vi "SwerveKinematics.vi"(0 "Joystick X":dbl(slide) scale=-1.0..1.0, 2 "Saturation Velocity (ul)":dbl=1.0, 5 "Joystick Y":dbl(slide) scale=1.0..-1.0, 7 "Joystick Rotation":dbl(slide) scale=1.0..-1.0, 9 "Cx (in)":dbl, 11 "Cy (in)":dbl) -> (1 "Module 0 Angle (deg)":dbl(knob) scale=180.0..-180.0 scale format="%#_6f", 3 "Module 1 Angle (deg)":dbl(knob) scale=180.0..-180.0 scale format="%#_6f", 4 "Module 0 Velocity Command (ul)":dbl(slide) scale=0.0..1.0 scale format="%.2f", 6 "Module 1 Velocity Command (ul)":dbl(slide) scale=0.0..1.0 scale format="%.2f", 10 "Module 2 Velocity Command (ul)":dbl(slide) scale=0.0..1.0 scale format="%.2f", 12 "Module 3 Angle (deg)":dbl(knob) scale=180.0..-180.0 scale format="%#_6f", 14 "Module 2 Angle (deg)":dbl(knob) scale=180.0..-180.0 scale format="%#_6f", 15 "Module 3 Velocity Command (ul)":dbl(slide) scale=0.0..1.0 scale format="%.2f")   [LabVIEW 2020]
doc: "Performs the kinematics for a rectangular four wheel swerve robot with a selectable center of rotation. Swerve module #0 is located in the front right corner and the modules increment in the counter-clockwise direction. This VI also handles de-saturating the drive velocity commands."
uses:
  GlobalDrivebase.vi
panel:
  # "\"Front\" of Robot"
  # "M1"
  # "M0"
  # "Left Thumbstick"
  # "Right Thumbstick"
  # "X"
  # "Y"
  # "(0,0)"
  # "+CCW"
  # "M2"
  # "M3"
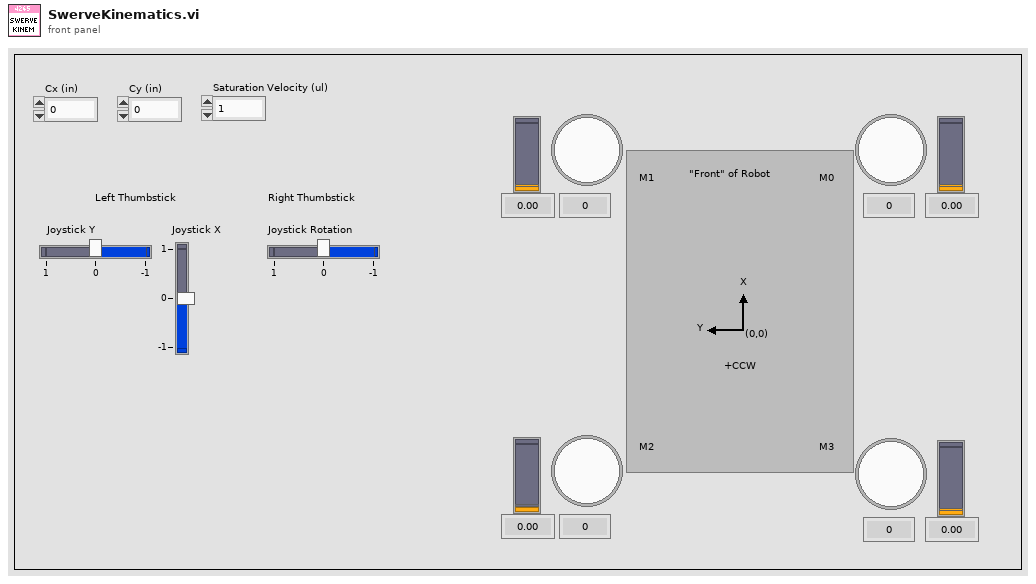
[diagram p1: front panel]
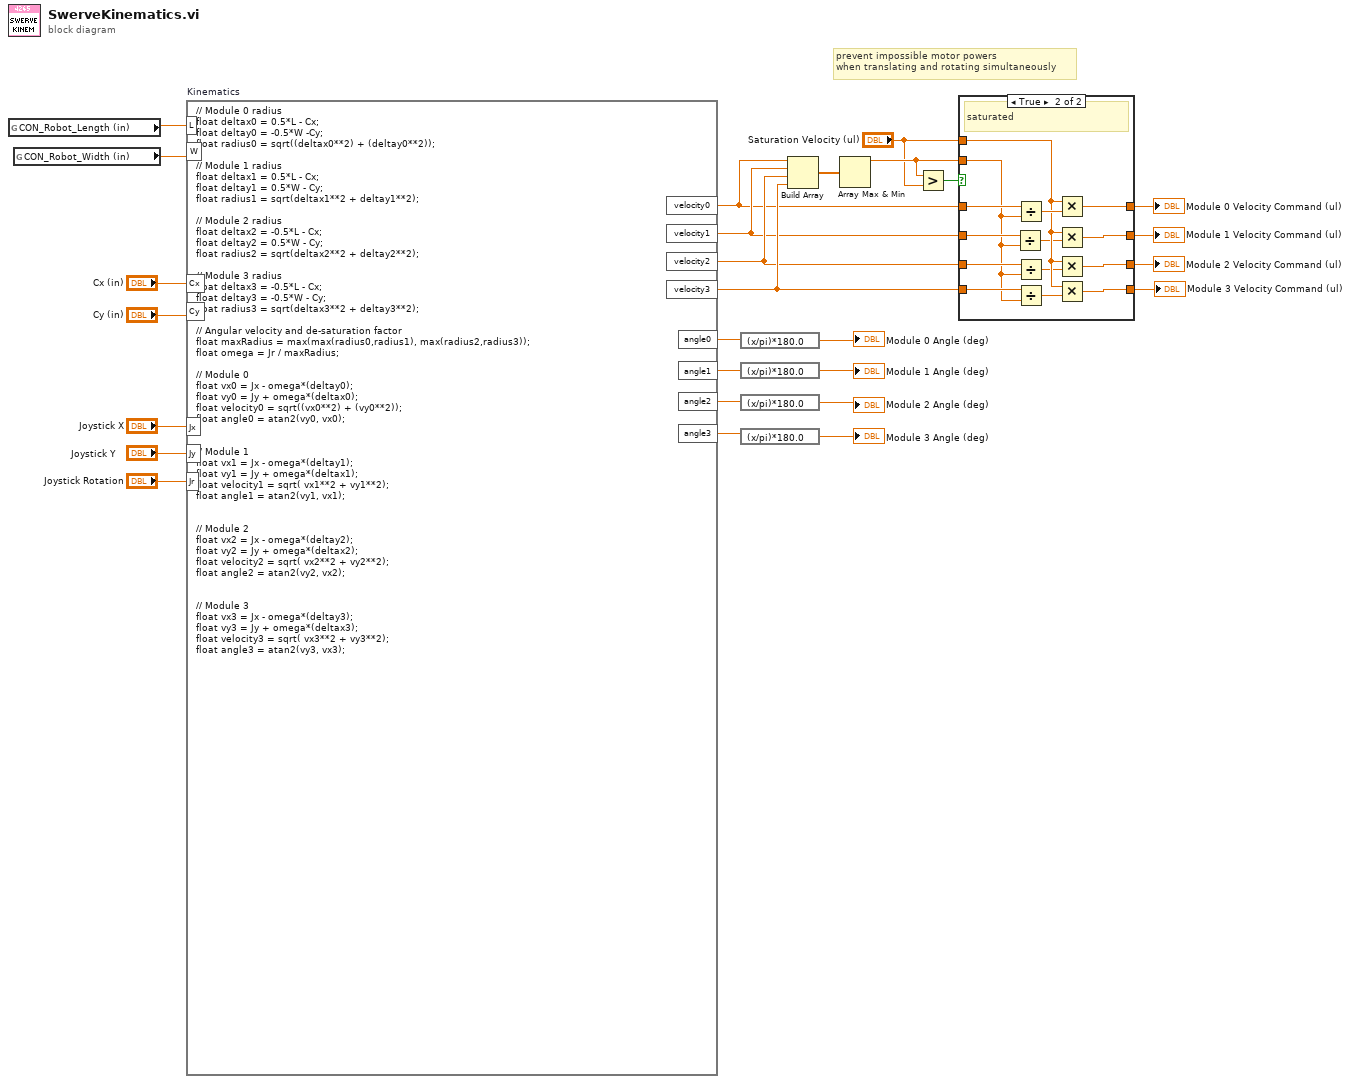
[diagram p0: block diagram]
diagram:
  # "prevent impossible motor powers\nwhen translating and rotating simultaneously"
  n1 = global read "GlobalDrivebase.vi" "CON_Robot_Length (in)"() -> (w2:dbl)
  n2 = global read "GlobalDrivebase.vi" "CON_Robot_Width (in)"() -> (w1:dbl)
  n3 = formula code="// Module 0 radius\nfloat deltax0 = 0.5*L - Cx;\nfloat deltay0 = -0.5*W -Cy; \nfloat radius0 = sqrt((deltax0**2) + (deltay0**2));\n\n// Module 1 radius\nfloat deltax1 = 0.5*L - Cx;\nfloat deltay1 = 0.5*W - Cy;\nfloat radius1 = sqrt(deltax1**2 + deltay1**2);\n\n// Module 2 radius\nfloat deltax2 = -0.5*L - Cx;\nfloat deltay2 = 0.5*W - Cy;\nfloat radius2 = sqrt(deltax2**2 + deltay2**2);\n\n// Module 3 radius\nfloat deltax3 = -0.5*L - Cx;\nfloat deltay3 = -0.5*W - Cy;\nfloat radius3 = sqrt(deltax3**2 + deltay3**2);\n\n// Angular velocity and de-saturation factor\nfloat maxRadius = max(max(radius0,radius1), max(radius2,radius3));\nfloat omega = Jr / maxRadius;\n\n// Module 0\nfloat vx0 = Jx - omega*(deltay0);\nfloat vy0 = Jy + omega*(deltax0);\nfloat velocity0 = sqrt((vx0**2) + (vy0**2));\nfloat angle0 = atan2(vy0, vx0);\n\n\n// Module 1\nfloat vx1 = Jx - omega*(deltay1);\nfloat vy1 = Jy + omega*(deltax1);\nfloat velocity1 = sqrt( vx1**2 + vy1**2);\nfloat angle1 = atan2(vy1, vx1);\n\n\n// Module 2\nfloat vx2 = Jx - omega*(deltay2);\nfloat vy2 = Jy + omega*(deltax2);\nfloat velocity2 = sqrt( vx2**2 + vy2**2);\nfloat angle2 = atan2(vy2, vx2);\n\n\n// Module 3\nfloat vx3 = Jx - omega*(deltay3);\nfloat vy3 = Jy + omega*(deltax3);\nfloat velocity3 = sqrt( vx3**2 + vy3**2);\nfloat angle3 = atan2(vy3, vx3);" "Kinematics"("L"=w2, "W"=w1, "Cx"="Cx (in)", "Cy"="Cy (in)", "Jr"="Joystick Rotation", "Jx"="Joystick X", "Jy"="Joystick Y") -> ("velocity0"=w16:dbl, "angle0"=w25:dbl, "angle1"=w23:dbl, "angle2"=w22:dbl, "angle3"=w21:dbl, "velocity1"=w17:dbl, "velocity2"=w18:dbl, "velocity3"=w19:dbl)
  n4 = expression code="(x/pi)*180.0" ("radians to degrees")(w25) -> (→"Module 0 Angle (deg)":dbl)
  n5 = expression code="(x/pi)*180.0" ("radians to degrees")(w23) -> (→"Module 1 Angle (deg)":dbl)
  n6 = expression code="(x/pi)*180.0" ("radians to degrees")(w22) -> (→"Module 2 Angle (deg)":dbl)
  n7 = expression code="(x/pi)*180.0" ("radians to degrees")(w21) -> (→"Module 3 Angle (deg)":dbl)
  n8 = Build Array(w16, w17, w18, w19) -> (w20:dbl[])
  n9 = Array Max & Min(array=w20) -> (max value=w5:dbl)  [unwired: 3 out]
  n10 = Greater?(x=w5, y="Saturation Velocity (ul)") -> (0:w3:bool)
  n11 = case shown="True" w3 {
    tunnel: w19 -> [w28 w45]
    tunnel: w18 -> [w29 w44]
    tunnel: w17 -> [w30 w43]
    tunnel: w16 -> [w31 w42]
    tunnel: [w31 w40] -> w14
    tunnel: [w30 w34] -> w12
    tunnel: [w29 w33] -> w10
    tunnel: [w28 w32] -> w8
    tunnel: w5 -> [_ w41]
    tunnel: "Saturation Velocity (ul)" -> [_ w38]
    frame False {
      # "not saturated"
    }
    frame True {
      # "saturated"
      n12 = Divide(x=w43, y=w41) -> (x/y=w35:dbl)
      n13 = Divide(x=w42, y=w41) -> (x/y=w39:dbl)
      n14 = Divide(x=w44, y=w41) -> (x/y=w37:dbl)
      n15 = Divide(x=w45, y=w41) -> (x/y=w36:dbl)
      n16 = Multiply(x=w38, y=w39) -> (x*y=w40:dbl)
      n17 = Multiply(x=w38, y=w35) -> (x*y=w34:dbl)
      n18 = Multiply(x=w38, y=w37) -> (x*y=w33:dbl)
      n19 = Multiply(x=w38, y=w36) -> (x*y=w32:dbl)
    }
  }
  "Module 0 Velocity Command (ul)" <- w14
  "Module 1 Velocity Command (ul)" <- w12
  "Module 2 Velocity Command (ul)" <- w10
  "Module 3 Velocity Command (ul)" <- w8
